vi "运维调试_氨氮.vi"() -> ()   [LabVIEW 2016, in "氨氮.lvlib"]
uses:
  <vilib>/Platform/TimedLoop/XDataNode/timing_clust.ctl
  <vilib>/Platform/TimedLoop/XDataNode/nitl_modes.ctl
  <vilib>/Platform/TimedLoop/XDataNode/wakeup.ctl
  <vilib>/Utility/miscctls.llb/LVPointTypeDef.ctl
  <vilib>/Platform/TimedLoop/XDataNode/XDataNode.xnode
  <vilib>/Platform/TimedLoop/XDataNode/XDNodeRunTimeDep.lvlib
panel:
  out "固件版本号":string
  in  "数组":string[](array[string])
  in  "备用系数写入":bool
  in  "备用系数读取":bool
  in  "备用系数":T1
  in  "量程切换阈值写入":bool
  in  "量程切换阈值读取":bool
  in  "量程切换阈值":cluster{"阈值":dbl, "标液浓度":dbl}
  in  "参数下拉列表":enum16{"氨氮", "总磷"}(ring)
  in  "量程下拉列表":enum16{"低量程", "高量程"}(ring)
  in  "测量模式下拉列表":enum16{"水样测量", "空白核查", "标样核查", "盲样测试", "加标回收"}(ring)
  in  "公式":cluster{"X^2":dbl, "X":dbl, "b":dbl}
  in  "写公式":bool
  in  "读公式":bool
  in  "精度":dbl=4.0
  in  "样品5 F0":dbl
  in  "样品5 F1":dbl
  in  "样品4 F1":dbl
  in  "样品4 F0":dbl
  in  "样品3 F0":dbl
  in  "样品3 F1":dbl
  in  "样品2 F0":dbl
  in  "样品2 F1":dbl
  in  "样品1 F1":dbl
  in  "样品1 F0":dbl
  in  "method":u16(ring) items=["最小二乘", "最小绝对残差", "Bisquare"]
  in  "模型":enum32{"线性", "多项式"}(ring)
  out "r^2":dbl format="%.7g"
  out "拟合公式":string
  in  "样品2启用":bool
  in  "样品5启用":bool
  in  "样品4启用":bool
  in  "样品3启用":bool
  in  "样品1启用":bool
  in  "标液浓度5":dbl
  out "测量吸光度5":dbl
  in  "标液浓度4":dbl
  out "测量吸光度4":dbl
  in  "标液浓度3":dbl
  out "测量吸光度3":dbl
  in  "标液浓度2":dbl
  out "测量吸光度2":dbl
  out "测量吸光度1":dbl
  in  "标液浓度1":dbl
  out "XY图":cluster{"X Values":dbl[], "Y Values":dbl[]}[](graph)
  in  "返回":bool
  in  "设置":bool
  out "序列号":string="序列号"
  out "氨氮测量数据":T2(xcontrol)
  out "集成报警信息":string
  out "设置值":dbl
  out "定时启动":bool
  out "总磷总氮运行状态":T3(xcontrol)
  in  "停止":bool
  in  "手动启动":bool
  in  "单步测试":bool
  in  "总磷氨氮调试":u16[](xcontrol)
  out "F3":sgl format="%#.6f"
  out "F2":sgl format="%#.6f"
  out "F1":sgl format="%#.6f"
  out "F0":sgl format="%#.6f"
  out "多列列表框":i32(listbox)
  # "COM7"
  # "参数设置"
  # "标液浓度"
  # "F0"
  # "F1"
  # "吸光值显示"
  # "样品一"
  # "辅\n助\n计\n算\n区"
  # "样品二"
  # "样品三"
  # "样品四"
  # "样品五"
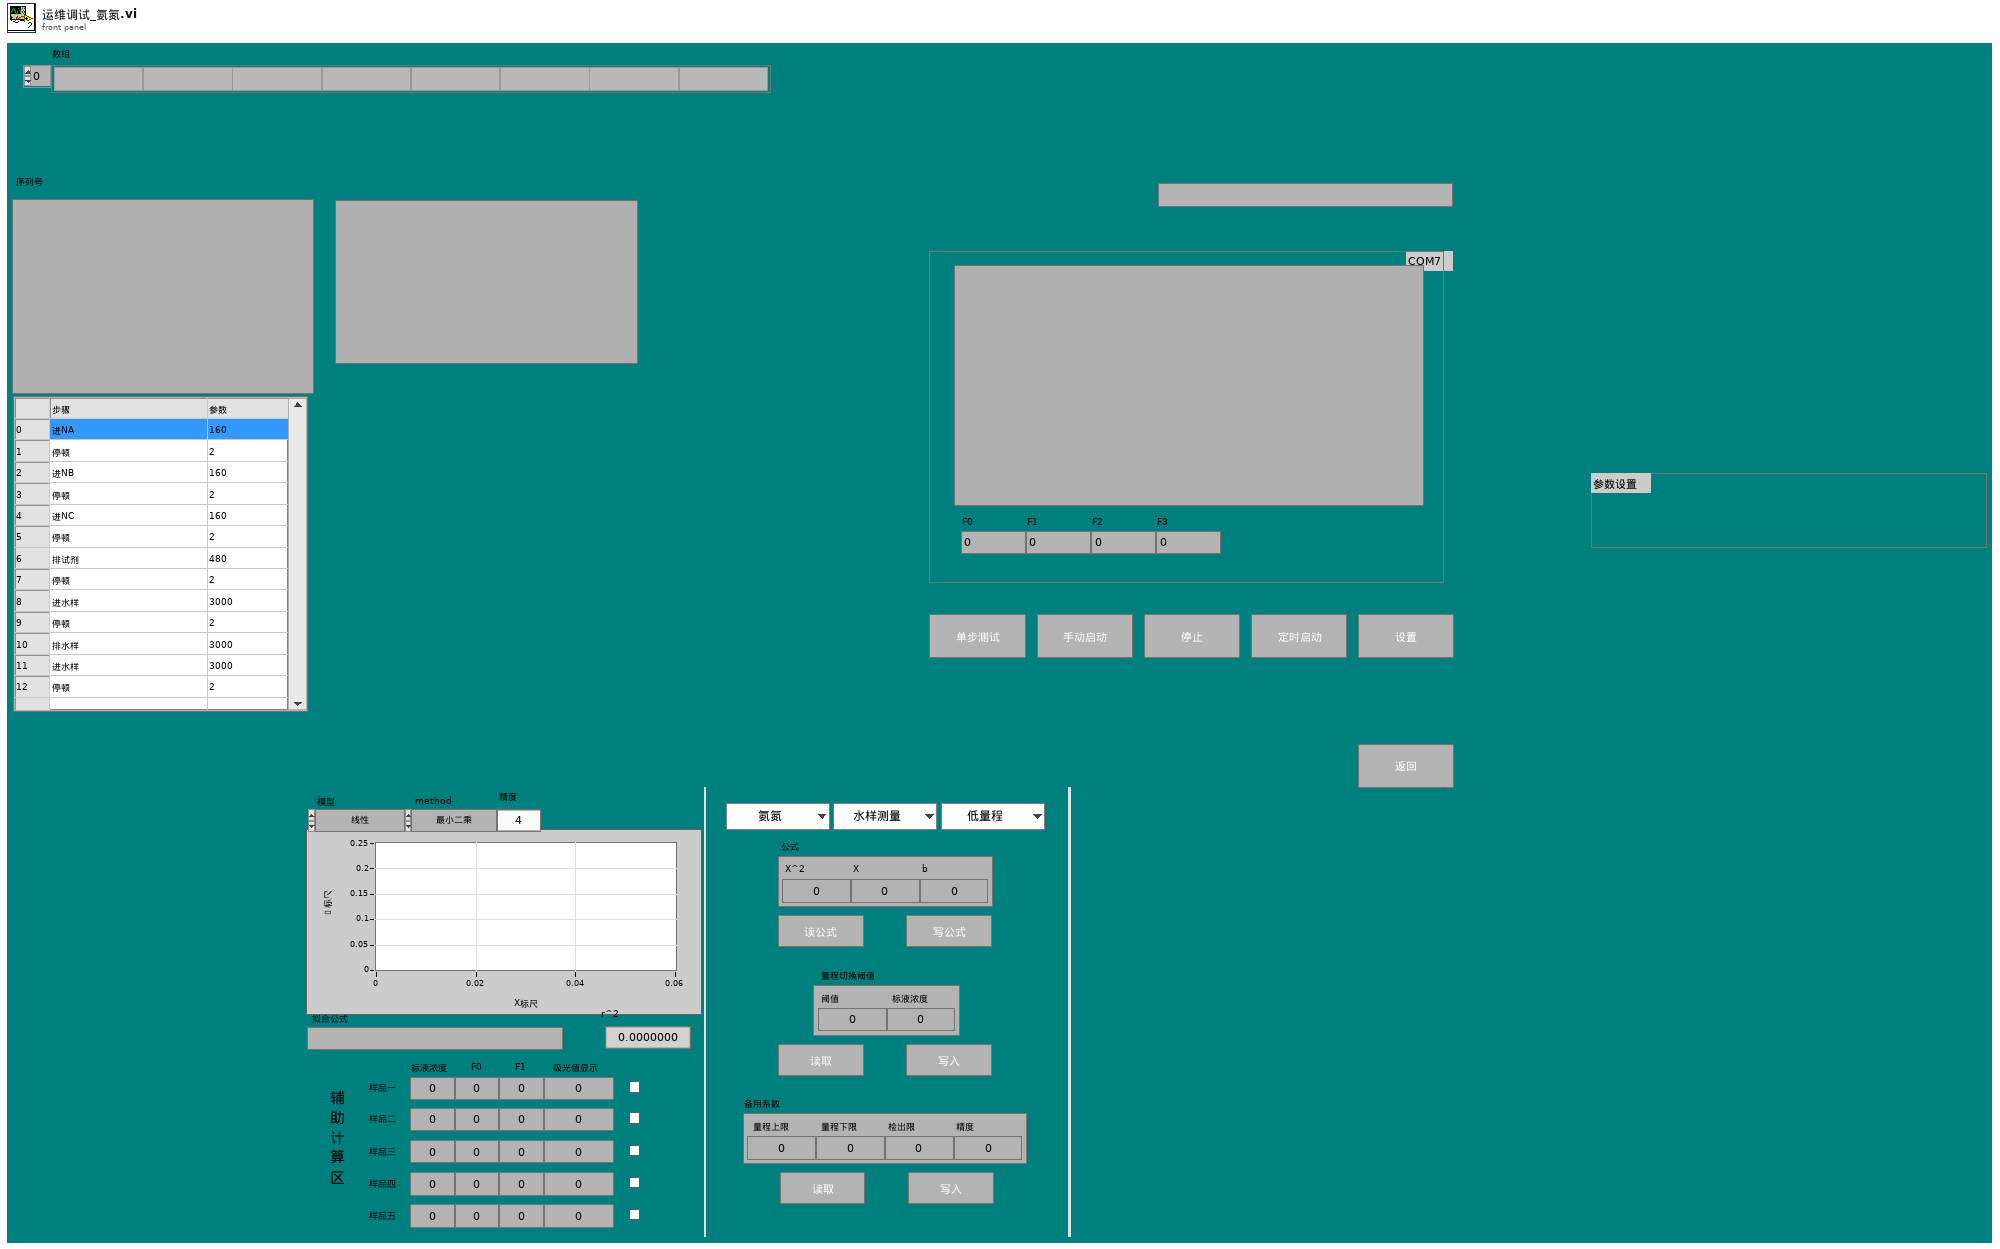
[diagram p1: front panel]
types:
  T1 = cluster{"量程上限":dbl, "量程下限":dbl, "检出限":dbl, "精度":dbl}
  T2 = cluster{"flowid":u16, "测量精度":u16, "测量数据区":cluster{"因子编码":u32, "单位":u16, "标样参考值":sgl, "水样数据时间":timestamp, "水样实测值":sgl, "水样数据标识":string, "标样数据时间":timestamp, "标样实测值":sgl, "标样数据标识":string, "空白数据时间":timestamp, "空白实测值":sgl, "空白数据标识":string, "零点核查数据时间":timestamp, "零点核查实测值":sgl, "零点核查数据标识":string, "跨度核查数据时间":timestamp, "跨度核查实测值":sgl, "跨度核查数据标识":string, "加标回收数据时间":timestamp, "加标回收实测值":sgl, "加标回收数据标识":string, "平行样数据时间":timestamp, "平行样实测值":sgl, "平行样数据标识":string}}
  T3 = cluster{"系统时间":timestamp, "工作状态":enum16{"空闲", "水样测试", "标样核查", "零点核查", "跨度核查", "空白测试", "平行样测试", "加标回收", "空白校准", "标样校准", "初始化（清洗）"}, "测量模式":enum16{"待机", "连续模式", "周期模式", "定点模式", "受控模式", "手动模式"}, "告警代码":enum16{"无告警", "缺试剂告警", "缺水样告警", "缺蒸馏水告警", "缺标液告警", "仪表漏液告警", "标定异常告警", "超量程告警", "加热异常", "低试剂预警", "超上限告警", "超下限告警", "仪表内部其他异常", "滴定异常告警", "电极异常告警", "量程切换告警", "参数设置告警", "PH电极电位异常", "电导率电极异常", "浊度光度异常", "溶解氧电极异常", "溶解氧光强异常", "温度异常告警", "PH异常告警", "溶解氧异常告警", "电导率异常告警", "浊度异常告警", "叶绿素异常告警", "藻密度异常告警", "蓝绿藻异常告警", "ORP异常告警", "氨氮异常告警", "清洁刷异常告警", "SD卡异常告警", "蓝牙异常告警", "Wifi异常告警", "流程异常告警"}, "故障代码":enum16{"无故障", "电机故障", "温度故障", "通讯故障", "滴定故障"}, "日志代码":u16, "软件版本":u16, "F0":sgl, "F1":sgl, "F2":sgl, "F3":sgl, "T":sgl, "H":sgl, "id":u16, "flowid":u16, "量程":u16}
  T4 = enum16{"待机", "启动氨氮", "氨氮测量中", "启动总磷", "总磷测量中", "延时"}
  T5 = typedef "LVPointTypeDef.ctl" = cluster{"Horizontal":i16, "Vertical":i16}
  T6 = cluster{"因子编码":u32, "单位":u16, "标样参考值":sgl, "水样数据时间":timestamp, "水样实测值":sgl, "水样数据标识":string, "标样数据时间":timestamp, "标样实测值":sgl, "标样数据标识":string, "空白数据时间":timestamp, "空白实测值":sgl, "空白数据标识":string, "零点核查数据时间":timestamp, "零点核查实测值":sgl, "零点核查数据标识":string, "跨度核查数据时间":timestamp, "跨度核查实测值":sgl, "跨度核查数据标识":string, "加标回收数据时间":timestamp, "加标回收实测值":sgl, "加标回收数据标识":string, "平行样数据时间":timestamp, "平行样实测值":sgl, "平行样数据标识":string}
  T7 = enum16{"空闲", "水样测试", "标样核查", "零点核查", "跨度核查", "空白测试", "平行样测试", "加标回收", "空白校准", "标样校准", "初始化（清洗）"}
  T8 = cluster{"启动模式":enum16{"标液测量", "水样测量", "零液测量", "盲样测量", "加标回收"}, "启动参数":u16, "量程":enum16{"低量程", "高量程"}}
  T9 = cluster{"时间标识":timestamp, "设备":string, "日志信息":string, "流程参数":string}
  T10 = cluster{"时间标识":timestamp, "设备":string, "日志信息":string}
  T11 = enum16{"无告警", "缺试剂告警", "缺水样告警", "缺蒸馏水告警", "缺标液告警", "仪表漏液告警", "标定异常告警", "超量程告警", "加热异常", "低试剂预警", "超上限告警", "超下限告警", "仪表内部其他异常", "滴定异常告警", "电极异常告警", "量程切换告警", "参数设置告警", "PH电极电位异常", "电导率电极异常", "浊度光度异常", "溶解氧电极异常", "溶解氧光强异常", "温度异常告警", "PH异常告警", "溶解氧异常告警", "电导率异常告警", "浊度异常告警", "叶绿素异常告警", "藻密度异常告警", "蓝绿藻异常告警", "ORP异常告警", "氨氮异常告警", "清洁刷异常告警", "SD卡异常告警", "蓝牙异常告警", "Wifi异常告警", "流程异常告警"}
  T12 = typedef "LVRowAndColumnUnsignedTypeDef.ctl" = cluster{"Row":u32, "Column":u32}
  T13 = typedef "XDNodeRunTimeDep.lvlib/timing_clust.ctl" = cluster{"Expected End [f-1]":u64, "Actual End [f-1]":u64, "Finished Late? [f-1]":bool, "Expected End [i-1]":u64, "Actual End [i-1]":u64, "Finished Late? [i-1]":bool, "Expected Start [i]":u64, "Actual Start [i]":u64, "Expected Start [f]":u64, "Actual Start [f]":u64, "Source Name":string, "Structure Name":string, "Period":i64, "Deadline":i64, "Offset":i64, "Start":i64, "Priority":i32, "Timeout":i32, "Mode":T14, "Wakeup Reason":T15, "Error":errorcluster, "Source Type":string, "Secondary Source Type":string, "Global End Time":u64, "Global Start Time":u64, "Frame Duration":u64, "Iteration Duration":u64, "Assigned CPU":i32, "I/O Scan Engine Mode":u32}
  T14 = typedef "XDNodeRunTimeDep.lvlib/nitl_modes.ctl" = enum32{"No Change", "Process missed periods, maintain original phase", "Discard missed periods, maintain original phase", "Process missed periods, ignore original phase", "Discard missed periods, ignore original phase"}
  T15 = typedef "XDNodeRunTimeDep.lvlib/wakeup.ctl" = enum32{"Normal", "Aborted", "Asynchronous wakeup", "Timing source error", "Timed loop error", "Timeout"}
  T16 = cluster{"站号":u16, "量程切换":enum32{"H", "L", "AUTO"}, "控制命令":enum16{"启动测量", "标样核查", "零点核查", "跨度核查", "空白测试", "平行样测试", "加标回收", "空白校准", "标样校准", "初始化（清洗）", "停止测试", "仪器重启", "校时", "模式设置", "测量间隔设置", "盲样测试"}, "模式设置":enum16{"待机", "连续模式", "周期模式", "定点模式", "受控模式", "手动模式"}, "测量间隔":u16}
  T17 = cluster{"站号":u16, "量程切换":enum32{"H", "L", "AUTO"}, "控制命令":enum16{"启动测量", "标样核查", "零点核查", "跨度核查", "空白测试", "平行样测试", "加标回收", "空白校准", "标样校准", "初始化（清洗）", "停止测试", "仪器重启", "校时", "模式设置", "测量间隔设置"}, "模式设置":enum16{"待机", "连续模式", "周期模式", "定点模式", "受控模式", "手动模式"}, "测量间隔":u16}
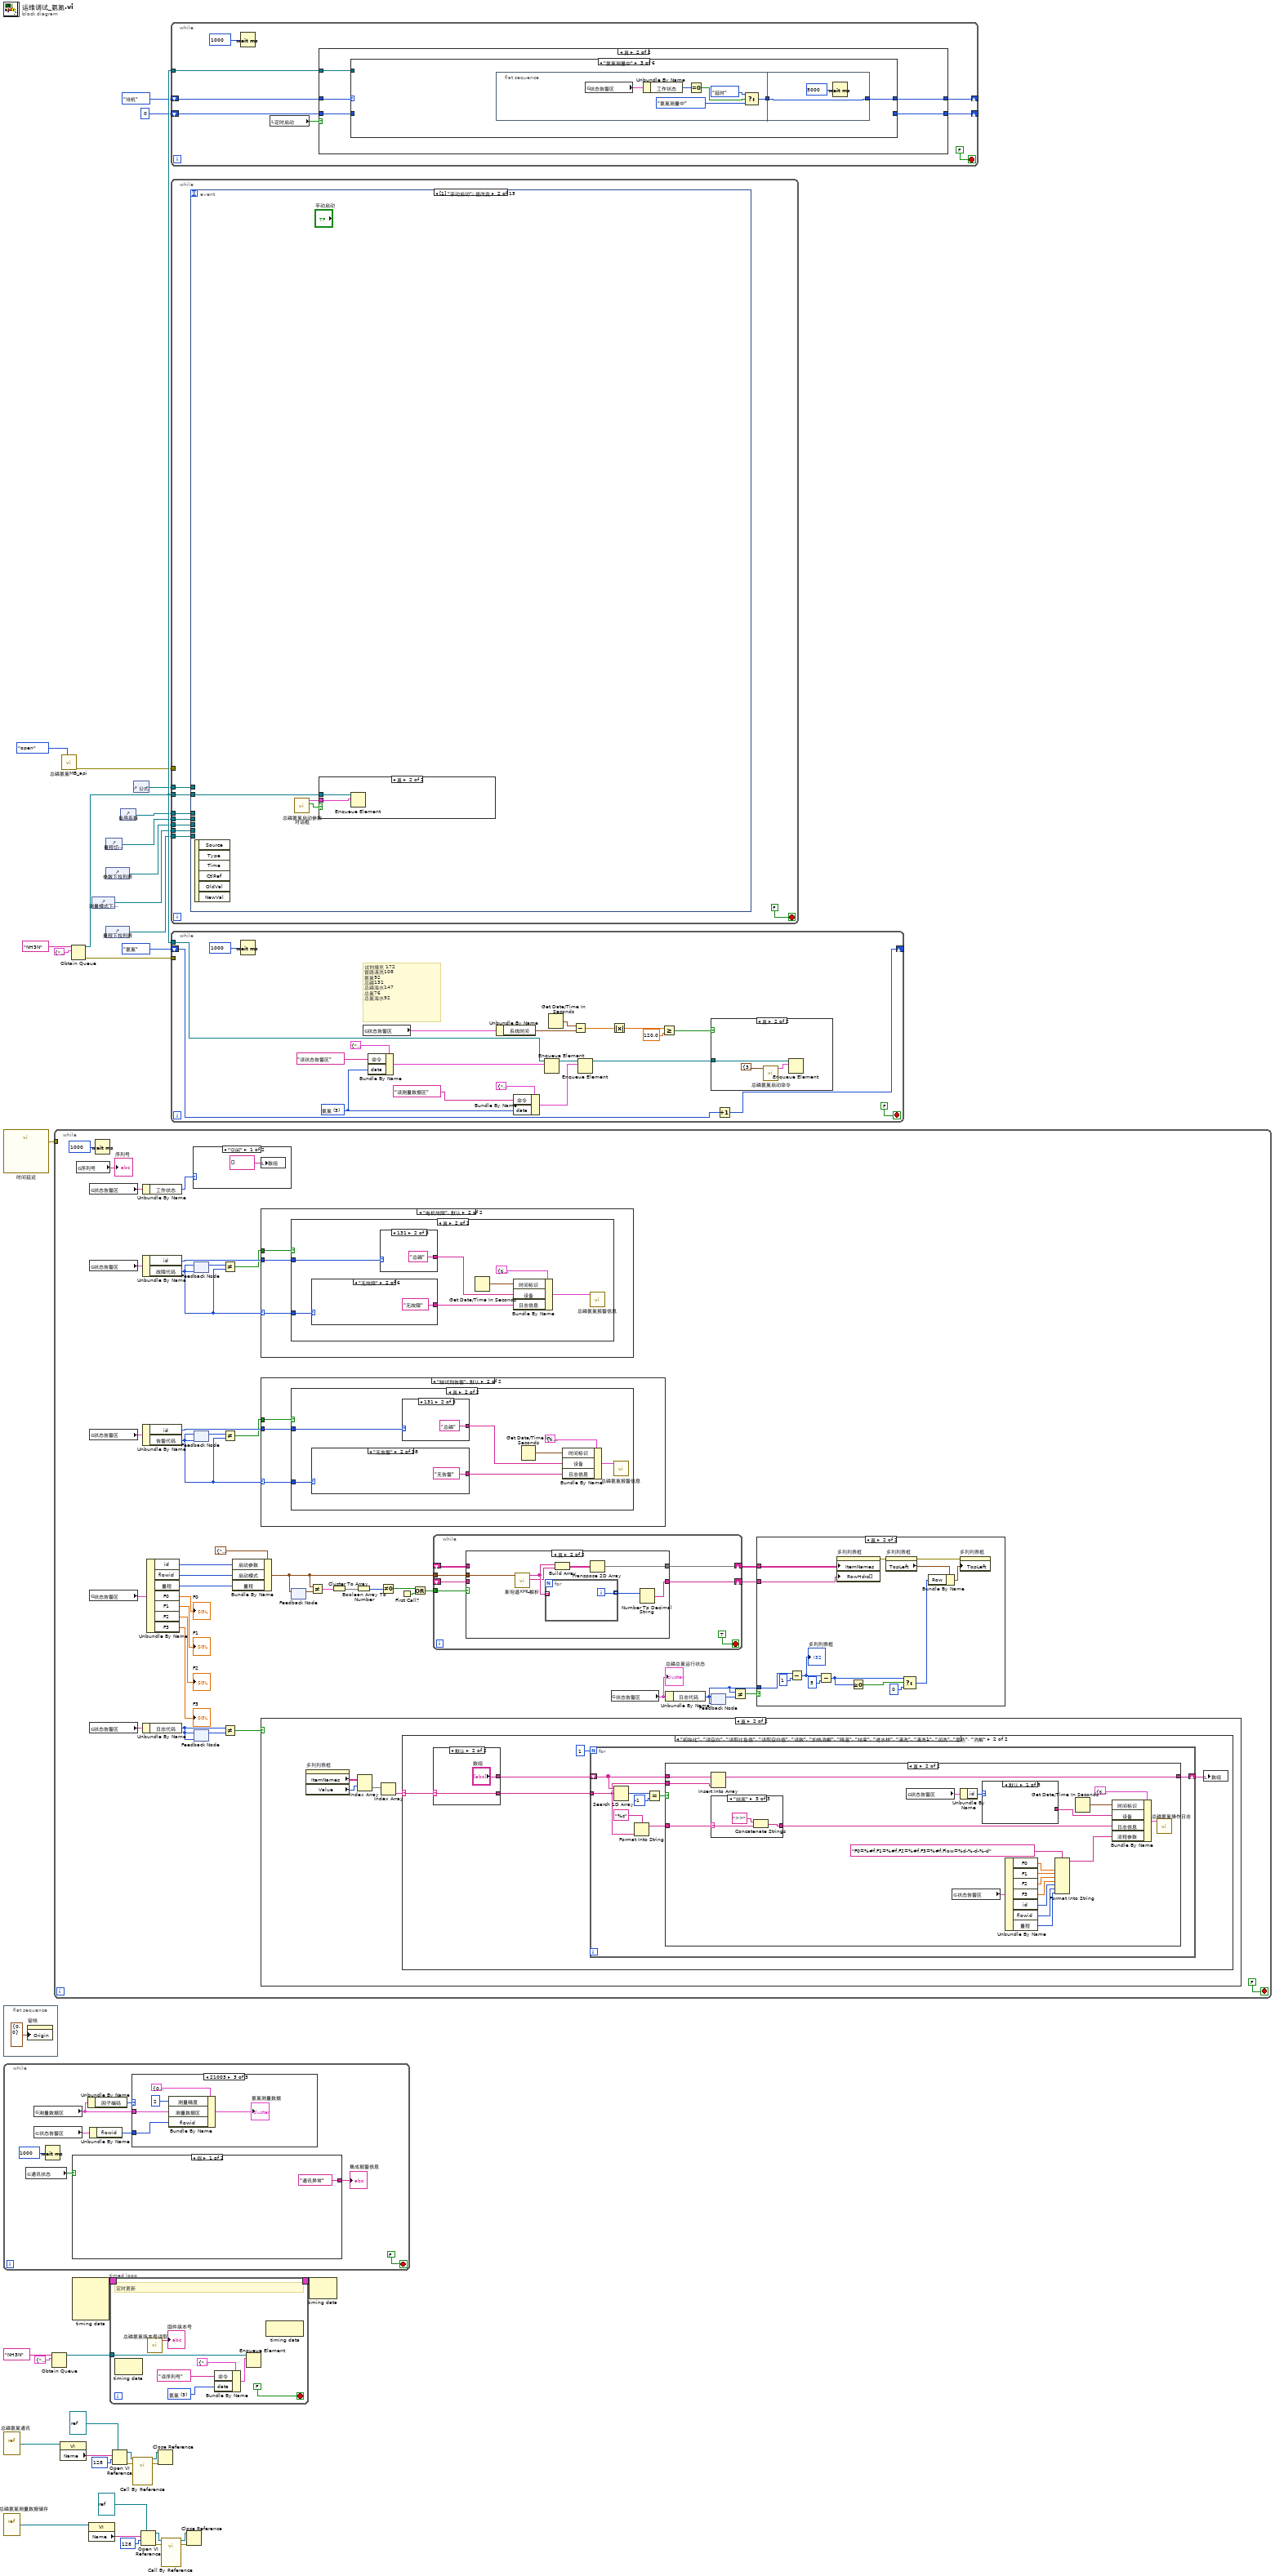
[diagram p0: block diagram]
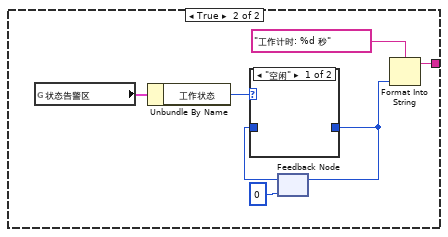
[diagram p2: hidden frame]
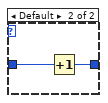
[diagram p3: hidden frame]
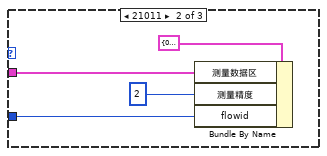
[diagram p5: hidden frame]
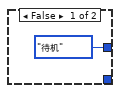
[diagram p6: hidden frame]
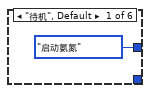
[diagram p7: hidden frame]
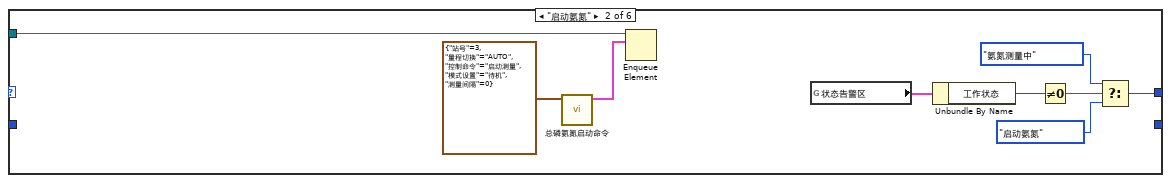
[diagram p8: hidden frame]
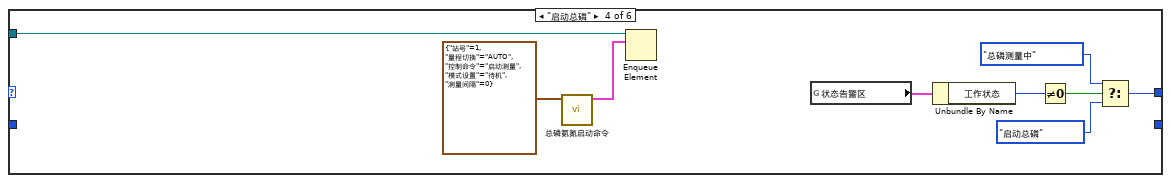
[diagram p9: hidden frame]
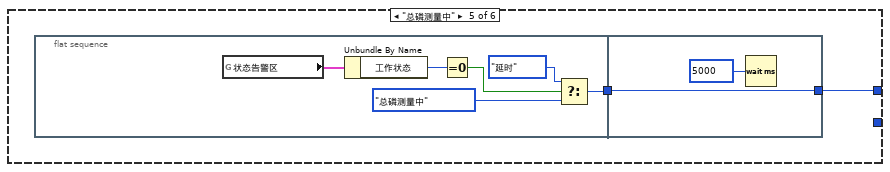
[diagram p10: hidden frame]
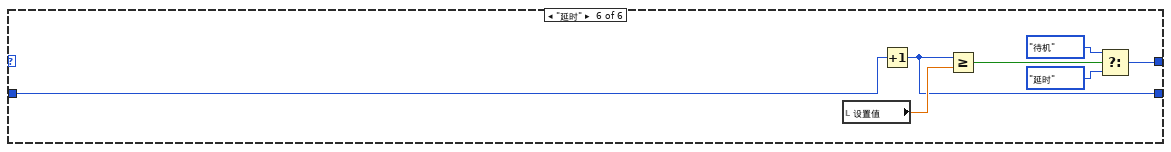
[diagram p11: hidden frame]
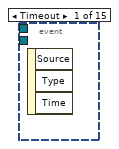
[diagram p12: hidden frame]
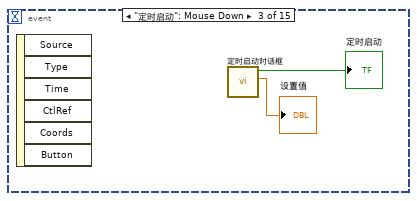
[diagram p14: hidden frame]
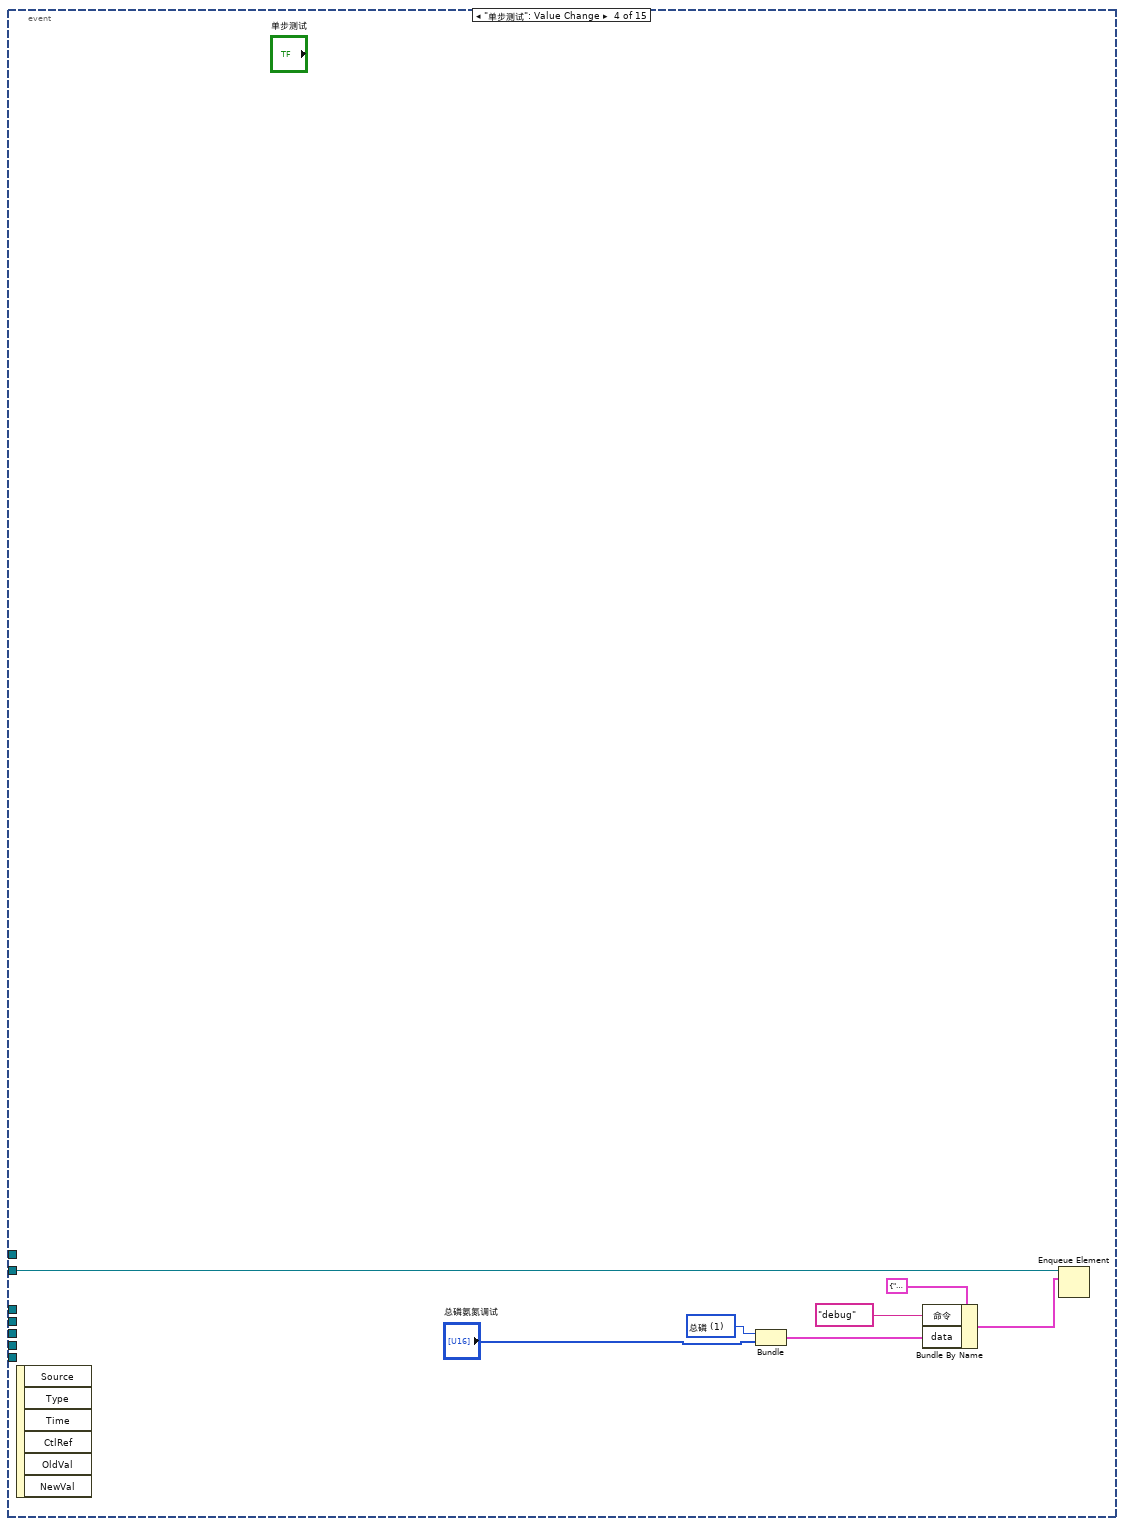
[diagram p15: hidden frame]
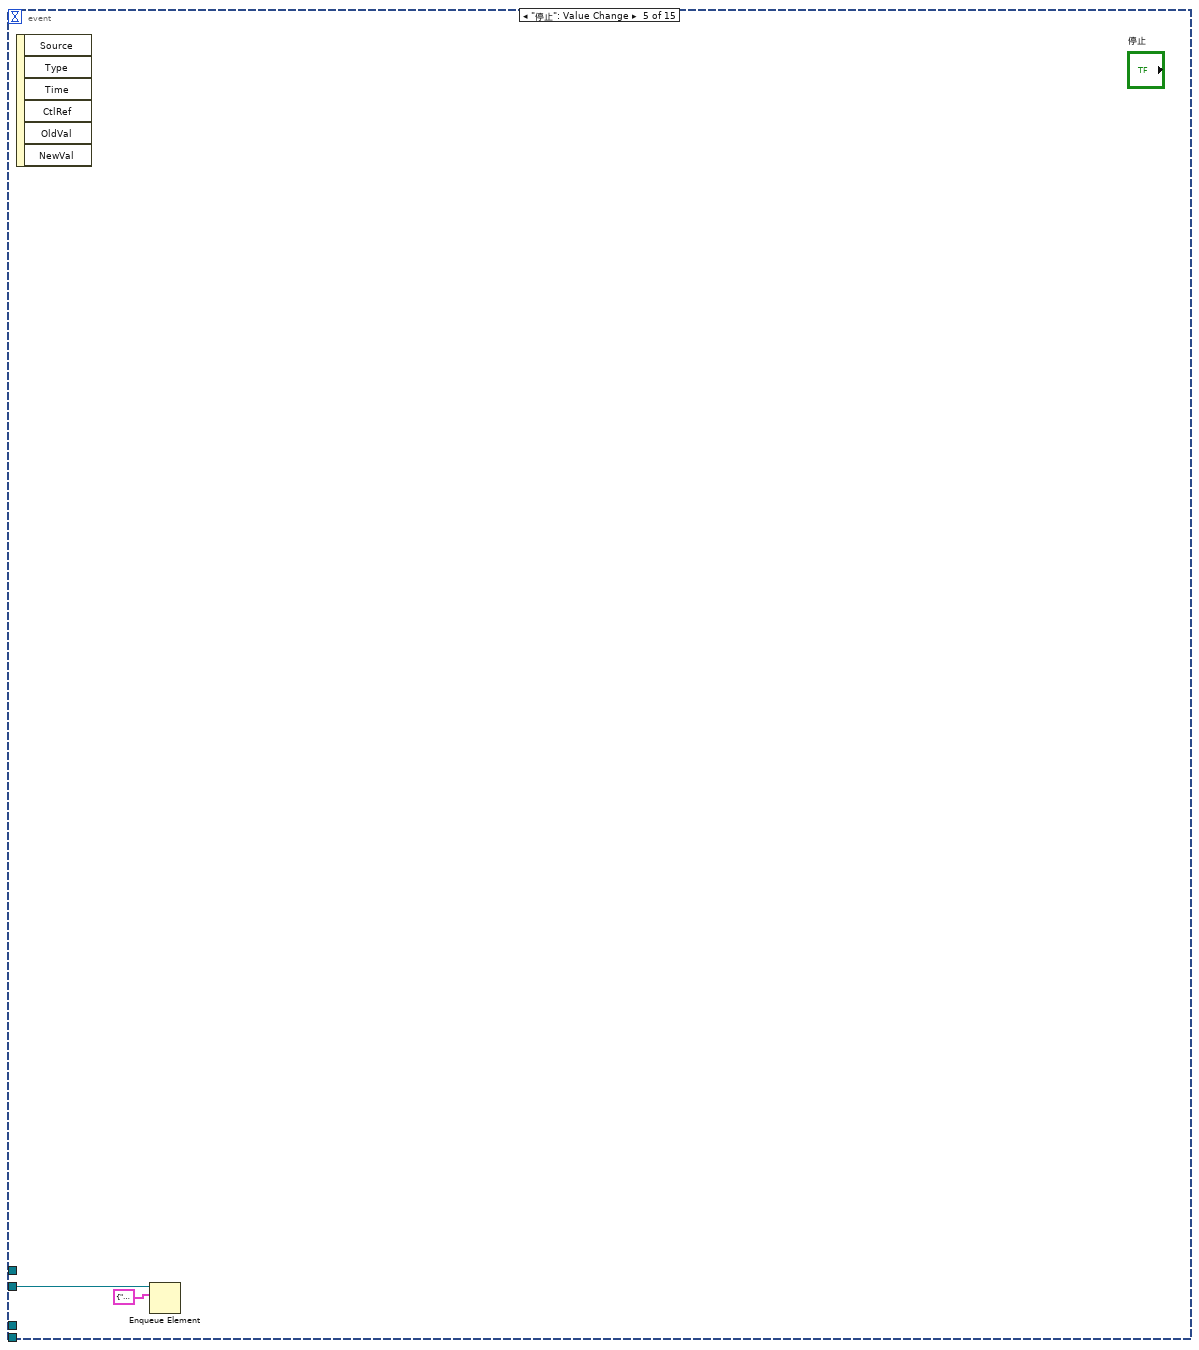
[diagram p16: hidden frame]
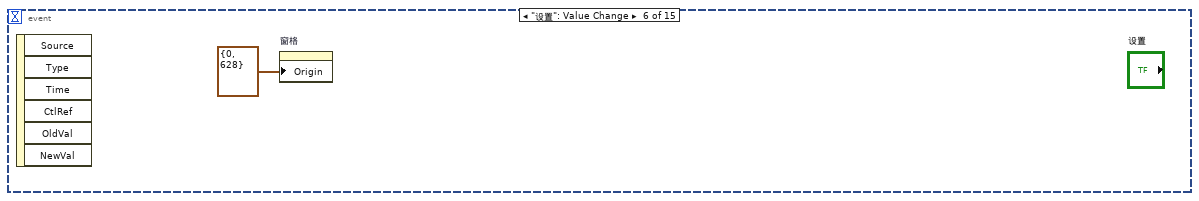
[diagram p17: hidden frame]
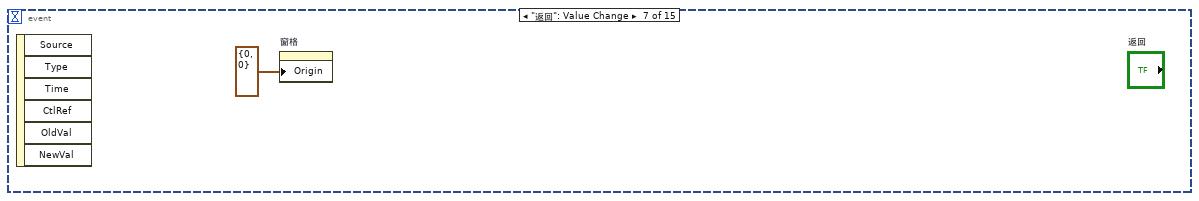
[diagram p18: hidden frame]
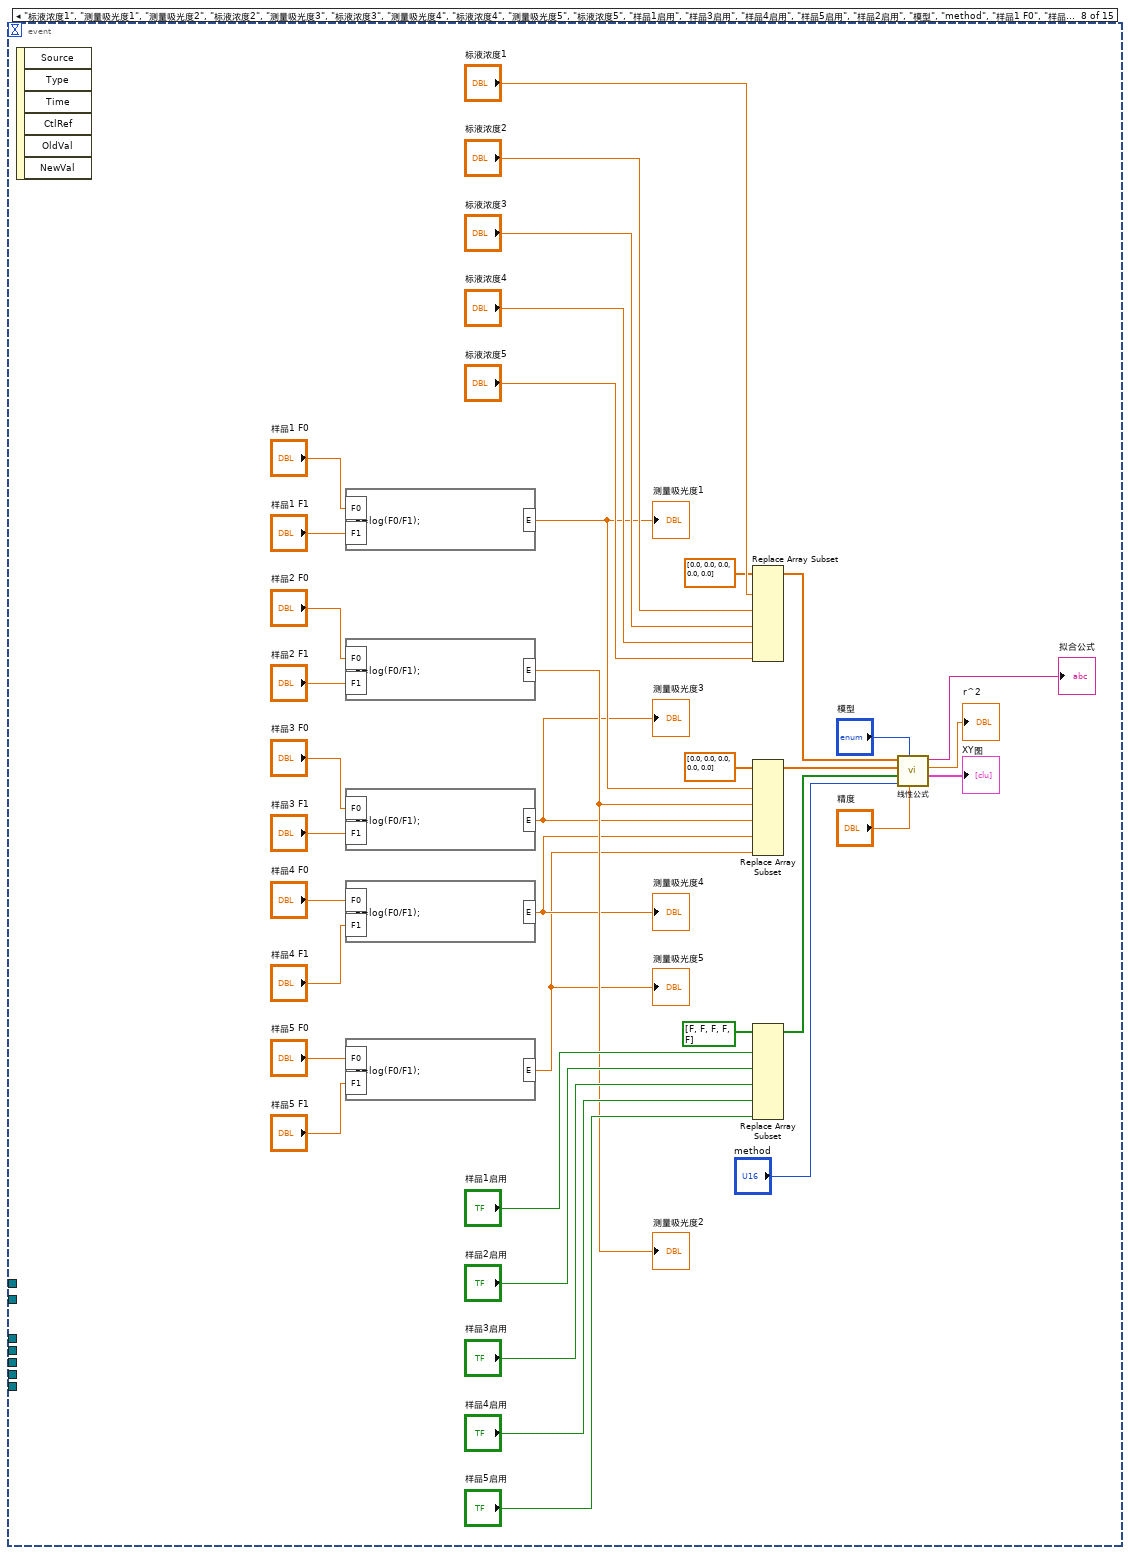
[diagram p19: hidden frame]
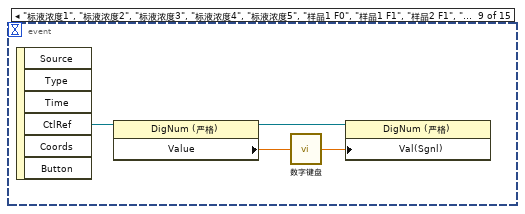
[diagram p20: hidden frame]
diagram:
  n1 = call "时间延迟"() -> ("error out"=w8:errorcluster)  [unwired: 11 in]
  n2 = flat-sequence {
    frame #0 {
      n3 = property on="窗格" class="Pane"("Origin"=T5 {"Horizontal"=0, "Vertical"=0} ("原点")) -> ()  [unwired: 2 in, 2 out]
    }
  }
  n4 = while {
    stop <- FALSE stop-if-true
    n5 = global read "VAR总磷氨氮全局变量.vi" "通讯状态"() -> (w42:bool)
    n6 = global read "VAR总磷氨氮全局变量.vi" "测量数据区"() -> (w44:T6)
    n7 = global read "VAR总磷氨氮全局变量.vi" "状态告警区"() -> (w40:T3)
    n8 = Wait (ms)(milliseconds to wait=u32 1000 ("等待时间（毫秒）")) -> ()  [unwired: 1 out]
    n9 = case shown="假" w42 {
      tunnel: ["通讯异常" ("集成报警信息") w48] -> w41
      frame False {
      }
      frame True {
        n10 = global read "VAR总磷氨氮全局变量.vi" "状态告警区"() -> (w54:T3)
        n11 = Unbundle By Name(w54) -> ("工作状态"=w53:T7)
        n12 = feedback #1(0) -> (w51:i32)
        n13 = case shown="\"空闲\"" w53 {
          tunnel: w51 -> [_ w56]
          tunnel: [_ w55] -> w49
          frame "空闲" {
          }
          frame Default {
            n14 = Increment(x=w56) -> (x+1=w55:i32)
          }
        }
        n15 = feedback-in #1(w49) -> ()
        n16 = Format Into String(format string="工作计时: %d 秒" ("格式字符串"), w49) -> (resulting string=w48:string)  [unwired: 2 in, 1 out]
      }
    }
    "集成报警信息" <- w41
    n17 = Unbundle By Name(w44) -> ("因子编码"=w43:u32)
    n18 = Unbundle By Name(w40) -> ("flowid"=w39:u16)
    n19 = case shown="21003" w43 {
      tunnel: w44 -> [_ w60 w65]
      tunnel: w39 -> [_ w58 w63]
      frame Default {
      }
      frame 21011 {
        n20 = Bundle By Name(cluster=T2 {"flowid"=0, "测量精度"=0, "测量数据区"={"因子编码"=0, "单位"=0, "标样参考值"=0.0, "水样数据时间"=timestamp(0 s since 1904-01-01), "水样实测值"=0.0, "水样数据标识"="", "标样数据时间"=timestamp(0 s since 1904-01-01), "标样实测值"=0.0, "标样数据标识"="", "空白数据时间"=timestamp(0 s since 1904-01-01), "空白实测值"=0.0, "空白数据标识"="", "零点核查数据时间"=timestamp(0 s since 1904-01-01), "零点核查实测值"=0.0, "零点核查数据标识"="", "跨度核查数据时间"=timestamp(0 s since 1904-01-01), "跨度核查实测值"=0.0, "跨度核查数据标识"="", "加标回收数据时间"=timestamp(0 s since 1904-01-01), "加标回收实测值"=0.0, "加标回收数据标识"="", "平行样数据时间"=timestamp(0 s since 1904-01-01), "平行样实测值"=0.0, "平行样数据标识"=""}} ("氨氮测量数据"), "测量数据区"=w60, "测量精度"=u16 2, "flowid"=w58) -> ()  [unwired: 1 out]
      }
      frame 21003 {
        n21 = Bundle By Name(cluster=T2 {"flowid"=0, "测量精度"=0, "测量数据区"={"因子编码"=0, "单位"=0, "标样参考值"=0.0, "水样数据时间"=timestamp(0 s since 1904-01-01), "水样实测值"=0.0, "水样数据标识"="", "标样数据时间"=timestamp(0 s since 1904-01-01), "标样实测值"=0.0, "标样数据标识"="", "空白数据时间"=timestamp(0 s since 1904-01-01), "空白实测值"=0.0, "空白数据标识"="", "零点核查数据时间"=timestamp(0 s since 1904-01-01), "零点核查实测值"=0.0, "零点核查数据标识"="", "跨度核查数据时间"=timestamp(0 s since 1904-01-01), "跨度核查实测值"=0.0, "跨度核查数据标识"="", "加标回收数据时间"=timestamp(0 s since 1904-01-01), "加标回收实测值"=0.0, "加标回收数据标识"="", "平行样数据时间"=timestamp(0 s since 1904-01-01), "平行样实测值"=0.0, "平行样数据标识"=""}} ("氨氮测量数据"), "测量精度"=u16 2, "测量数据区"=w65, "flowid"=w63) -> (→"氨氮测量数据":T2)
      }
    }
  }
  n22 = vi-ref "总磷氨氮通讯.vi"() -> (w31:refnum<vi>)
  n23 = vi-ref "总磷氨氮测量数据储存.vi"() -> (w23:refnum<vi>)
  n24 = Obtain Queue(name (unnamed)="NH3N" ("名称（未命名）"), element data type=cluster{"命令":string, "data":variant} {"命令"="", "data"=variant}) -> (queue out=w1:refnum<queue>)  [unwired: 3 in, 2 out]
  n25 = while {
    tunnel: w8 -> [_]
    stop <- FALSE stop-if-true
    n26 = global read "VAR总磷氨氮全局变量.vi" "序列号"() -> (→"序列号":string)
    n27 = global read "VAR总磷氨氮全局变量.vi" "状态告警区"() -> (w71:T3)
    n28 = global read "VAR总磷氨氮全局变量.vi" "状态告警区"() -> (w77:T3)
    n29 = global read "VAR总磷氨氮全局变量.vi" "状态告警区"() -> (w82:T3)
    n30 = global read "VAR总磷氨氮全局变量.vi" "状态告警区"() -> (w94:T3)
    n31 = global read "VAR总磷氨氮全局变量.vi" "状态告警区"() -> (w68:T3)
    n32 = Wait (ms)(milliseconds to wait=u32 1000 ("等待时间（毫秒）")) -> ()  [unwired: 1 out]
    n33 = Unbundle By Name(w71) -> ("工作状态"=w70:T7)
    n34 = Unbundle By Name(w77) -> ("id"=w76:u16, "故障代码"=w73:enum16{"无故障", "电机故障", "温度故障", "通讯故障", "滴定故障"})
    n35 = Unbundle By Name(w82) -> ("id"=w81:u16, "告警代码"=w78:T11)
    n36 = Unbundle By Name(w68) -> ("日志代码"=w67:u16)
    n37 = Unbundle By Name(w94) -> ("id"=w91:u16, "flowid"=w93:u16, "量程"=w92:u16, "F0"=→"F0":sgl, "F1"=→"F1":sgl, "F2"=→"F2":sgl, "F3"=→"F3":sgl)
    n38 = case shown="\"空闲\"" w70 {
      frame "空闲" {
        n39 = local write "数组"(string[] [] ("数组")) -> ()
      }
      frame "水样测试", Default {
      }
    }
    n40 = feedback #2(w73) -> (w74:enum16{"无故障", "电机故障", "温度故障", "通讯故障", "滴定故障"})
    n41 = feedback-in #2(w73) -> ()
    n42 = feedback #3(w78) -> (w79:T11)
    n43 = feedback-in #3(w78) -> ()
    n44 = feedback #4(w67) -> (w69:u16)
    n45 = feedback-in #4(w67) -> ()
    n46 = Not Equal?(x=w74, y=w73) -> (x != y?=w75:bool)
    n47 = Not Equal?(x=w79, y=w78) -> (x != y?=w80:bool)
    n48 = Not Equal?(x=w67, y=w69) -> (x != y?=w66:bool)
    n49 = Bundle By Name(cluster=T8 {"启动模式"=enum."加标回收", "启动参数"=1, "量程"=enum."低量程"} ("参数簇"), "启动参数"=w91, "启动模式"=w93, "量程"=w92) -> (w84:T8)
    n50 = case shown="\"电机故障\", 默认" w73 {
      selector: w73 -> [_ w162]
      tunnel: w76 -> [_ w163]
      tunnel: w75 -> [_ w161]
      frame "无故障" {
      }
      frame "电机故障", Default {
        n51 = case shown="真" w161 {
          tunnel: w163 -> [_ w170]
          tunnel: w162 -> [_ w165]
          frame False {
          }
          frame True {
            n52 = case shown="\"无故障\"" w165 {
              selector: w165 -> [w172 _ _ _ _ _]
              tunnel: [w171 "无故障" "电机故障" "温度故障" "通讯故障" "滴定故障"] -> w164
              frame Default {
                n53 = Format Into String(format string="%d" ("格式字符串"), initial string="未知" ("工作状态"), w172) -> (resulting string=w171:string)  [unwired: 1 in, 1 out]
              }
              frame "无故障" {
              }
              frame "电机故障" {
              }
              frame "温度故障" {
              }
              frame "通讯故障" {
              }
              frame "滴定故障" {
              }
            }
            n54 = case shown="131" w170 {
              tunnel: [_ "总磷" ("table输入") "氨氮" ("table输入")] -> w166
              frame Default {
              }
              frame 131 {
              }
              frame 92 {
              }
            }
            n55 = Get Date/Time In Seconds() -> (seconds since 1Jan1904=w167:timestamp)
            n56 = Bundle By Name(cluster=T10 {"时间标识"=timestamp(0 s since 1904-01-01), "设备"="", "日志信息"=""} ("data in"), "时间标识"=w167, "设备"=w166, "日志信息"=w164) -> (w168:T10)
            n57 = call "总磷氨氮报警信息.vi"("data in"=w168) -> ()  [unwired: 11 in]
          }
        }
      }
    }
    n58 = case shown="\"缺试剂告警\", 默认" w78 {
      selector: w78 -> [_ w183]
      tunnel: w81 -> [_ w184]
      tunnel: w80 -> [_ w182]
      frame "无告警" {
      }
      frame "缺试剂告警", Default {
        n59 = case shown="真" w182 {
          tunnel: w184 -> [_ w191]
          tunnel: w183 -> [_ w185]
          frame False {
          }
          frame True {
            n60 = case shown="\"无告警\"" w185 {
              selector: w185 -> [w193 _ _ _ _ _ _ _ _ _ _ _ _ _ _ _ _ _ _ _ _ _ _ _ _ _ _ _ _ _ _ _ _ _ _ _ _ _]
              tunnel: [w192 "无告警" "缺试剂告警" "缺水样告警" "缺蒸馏水告警" "缺标液告警" "仪表漏液告警" "标定异常告警" "超量程告警" "加热异常" "低试剂预警" "超上限告警" "超下限告警" "仪表内部其他异常" "滴定异常告警" "电极异常告警" "量程切换告警" "参数设置告警" "PH电极电位异常" "电导率电极异常" "浊度光度异常" "溶解氧电极异常" "溶解氧光强异常" "温度异常告警" "PH异常告警" "溶解氧异常告警" "电导率异常告警" "浊度异常告警" "叶绿素异常告警" "藻密度异常告警" "蓝绿藻异常告警" "ORP异常告警" "氨氮异常告警" "清洁刷异常告警" "SD卡异常告警" "蓝牙异常告警" "WiFi异常告警" "流程异常告警"] -> w186
              frame Default {
                n61 = Format Into String(format string="%d" ("格式字符串"), initial string="未知" ("工作状态"), w193) -> (resulting string=w192:string)  [unwired: 1 in, 1 out]
              }
              frame "无告警" {
              }
              frame "缺试剂告警" {
              }
              frame "缺水样告警" {
              }
              frame "缺蒸馏水告警" {
              }
              frame "缺标液告警" {
              }
              frame "仪表漏液告警" {
              }
              frame "标定异常告警" {
              }
              frame "超量程告警" {
              }
              frame "加热异常" {
              }
              frame "低试剂预警" {
              }
              frame "超上限告警" {
              }
              frame "超下限告警" {
              }
              frame "仪表内部其他异常" {
              }
              frame "滴定异常告警" {
              }
              frame "电极异常告警" {
              }
              frame "量程切换告警" {
              }
              frame "参数设置告警" {
              }
              frame "PH电极电位异常" {
              }
              frame "电导率电极异常" {
              }
              frame "浊度光度异常" {
              }
              frame "溶解氧电极异常" {
              }
              frame "溶解氧光强异常" {
              }
              frame "温度异常告警" {
              }
              frame "PH异常告警" {
              }
              frame "溶解氧异常告警" {
              }
              frame "电导率异常告警" {
              }
              frame "浊度异常告警" {
              }
              frame "叶绿素异常告警" {
              }
              frame "藻密度异常告警" {
              }
              frame "蓝绿藻异常告警" {
              }
              frame "ORP异常告警" {
              }
              frame "氨氮异常告警" {
              }
              frame "清洁刷异常告警" {
              }
              frame "SD卡异常告警" {
              }
              frame "蓝牙异常告警" {
              }
              frame "Wifi异常告警" {
              }
              frame "流程异常告警" {
              }
            }
            n62 = case shown="131" w191 {
              tunnel: [_ "总磷" ("table输入") "氨氮" ("table输入")] -> w187
              frame Default {
              }
              frame 131 {
              }
              frame 92 {
              }
            }
            n63 = Get Date/Time In Seconds() -> (seconds since 1Jan1904=w188:timestamp)
            n64 = Bundle By Name(cluster=T10 {"时间标识"=timestamp(0 s since 1904-01-01), "设备"="", "日志信息"=""} ("data in"), "时间标识"=w188, "设备"=w187, "日志信息"=w186) -> (w189:T10)
            n65 = call "总磷氨氮报警信息.vi"("data in"=w189) -> ()  [unwired: 11 in]
          }
        }
      }
    }
    n66 = case shown="真" w66 {
      frame False {
      }
      frame True {
        n67 = property on="多列列表框" class="MCListbox (严格)"() -> ("ItemNames"=w111:string[][], "Value"=w112:i32)  [unwired: 2 in, 2 out]
        n68 = Index Array(array=w111, index (row)=w112) -> (element=w110:string[])  [unwired: 1 in]
        n69 = Index Array(array=w110) -> (element=w109:string)  [unwired: 1 in]
        n70 = case shown="\"初始化\", \"读空白\", \"读取比色值\", \"读取空白值\", \"读数\", \"加热消解\", \"降温\", \"结束\", \"进水样\", \"清洗\", \"清洗1\", \"润洗\", \"显色\", \"消解\"" w109 {
          selector: w109 -> [_ w115]
          frame Default {
          }
          frame "初始化", "读空白", "读取比色值", "读取空白值", "读数", "加热消解", "降温", "结束", "进水样", "清洗", "清洗1", "润洗", "显色", "消解" {
            n71 = case shown="默认" w115 {
              selector: w115 -> [w119 w121]
              tunnel: [w119 w121] -> w114
              tunnel: [string[] [] ("数组") "数组"] -> w113
              frame "读数" {
              }
              frame Default {
              }
            }
            n72 = for {
              N: 1 -> [_]
              tunnel: w114 -> [w123]
              shift-right: [w122] -> w116
              shift-left: w113 -> [w124]
              n73 = Search 1D Array(1D array=w124, element=w123) -> (index of element=w127:i32)  [unwired: 1 in]
              n74 = Format Into String(format string="%s" ("格式字符串"), w123) -> (resulting string=w128:string)  [unwired: 2 in, 1 out]
              n75 = Equal?(x=w127, y=-1) -> (x = y?=w125:bool)
              n76 = case shown="真" w125 {
                tunnel: w128 -> [_ w132]
                tunnel: w124 -> [w130 w136]
                tunnel: w123 -> [_ w135]
                tunnel: [w130 w134] -> w122
                frame False {
                }
                frame True {
                  n77 = Insert Into Array(array=w136, new element=w135) -> (w134:string[])  [unwired: 1 in]
                  n78 = case shown="\"结束\"" w132 {
                    selector: w132 -> [w152 w155 w158]
                    tunnel: [w152 w154 w157] -> w131
                    frame Default {
                    }
                    frame "初始化" {
                      n79 = Concatenate Strings("<<" ("字符串"), w155) -> (w154:string)
                    }
                    frame "结束" {
                      n80 = Concatenate Strings(">>" ("字符串"), w158) -> (w157:string)
                    }
                  }
                  n81 = global read "VAR总磷氨氮全局变量.vi" "状态告警区"() -> (w151:T3)
                  n82 = global read "VAR总磷氨氮全局变量.vi" "状态告警区"() -> (w146:T3)
                  n83 = Unbundle By Name(w151) -> ("id"=w150:u16)
                  n84 = case shown="默认" w150 {
                    tunnel: [_ "总磷" ("table输入") "氨氮" ("table输入")] -> w148
                    frame Default {
                    }
                    frame 131 {
                    }
                    frame 92 {
                    }
                  }
                  n85 = Unbundle By Name(w146) -> ("F0"=w143:sgl, "F1"=w142:sgl, "F2"=w141:sgl, "F3"=w140:sgl, "id"=w139:u16, "flowid"=w138:u16, "量程"=w137:u16)
                  n86 = Format Into String(format string="F0=%#f,F1=%#f,F2=%#f,F3=%#f,Flow=%d-%-d-%-d" ("格式字符串"), w143, w142, w141, w140, w139, w138, w137) -> (resulting string=w144:string)  [unwired: 2 in, 1 out]
                  n87 = Get Date/Time In Seconds() -> (seconds since 1Jan1904=w147:timestamp)
                  n88 = Bundle By Name(cluster=T9 {"时间标识"=timestamp(0 s since 1904-01-01), "设备"="", "日志信息"="", "流程参数"=""} ("data in"), "时间标识"=w147, "设备"=w148, "日志信息"=w131, "流程参数"=w144) -> (w149:T9)
                  n89 = call "总磷氨氮操作日志.vi"("data in"=w149) -> ()  [unwired: 11 in]
                }
              }
            }
            n90 = local write "数组"(w116) -> ()
          }
        }
      }
    }
    n91 = feedback #5() -> (w100:T8)  [unwired: 1 in]
    n92 = feedback-in #5(w84) -> ()
    n93 = Not Equal?(x=w84, y=w100) -> (x != y?=w101:cluster{"启动模式":bool, "启动参数":bool, "量程":bool})
    n94 = Cluster To Array(cluster=w101) -> (array=w102:bool[])
    n95 = Boolean Array To Number(Boolean array=w102) -> (number=w103:u32)
    n96 = Not Equal To 0?(x=w103) -> (x != 0?=w96:bool)
    n97 = First Call?() -> (First Call?: T/F=w97:bool)
    n98 = Or(x=w96, y=w97) -> (x .or. y?=w95:bool)
    n99 = while {
      tunnel: w95 -> [w241]
      tunnel: w84 -> [w240]
      shift-right: [w239] -> w99
      shift-left: _ -> [w235]
      shift-right: [w238] -> w98
      shift-left: _ -> [w236]
      stop <- TRUE stop-if-true
      n100 = case shown="真" w241 {
        tunnel: [w243 w250] -> w238
        tunnel: [w242 w249] -> w239
        tunnel: w240 -> [_ w244]
        tunnel: w236 -> [w243 _]
        tunnel: w235 -> [w242 _]
        frame False {
        }
        frame True {
          n101 = call "斯坦道XML解析.vi"("参数簇"=w244) -> ("步骤时间"=w245:string[], "步骤名"=w247:string[])  [unwired: 9 in]
          n102 = for {
            tunnel: w247 -> [_] mode=indexing
            tunnel: [w251] -> w248 mode=indexing
            i -> [w251]
          }
          n103 = Build Array(w247, w245) -> (w246:string[][])
          n104 = Transpose 2D Array(2D array=w246) -> (transposed array=w249:string[][])
          n105 = Number To Decimal String(number=w248) -> (decimal integer string=w250:string[])  [unwired: 1 in]
        }
      }
    }
    n106 = global read "VAR总磷氨氮全局变量.vi" "状态告警区"() -> (w85:T3)
    "总磷总氮运行状态" <- w85
    n107 = Unbundle By Name(w85) -> ("日志代码"=w72:u16)
    n108 = feedback-in #6(w72) -> ()
    n109 = feedback #6(w72) -> (w105:u16)
    n110 = Not Equal?(x=w72, y=w105) -> (x != y?=w104:bool)
    n111 = case shown="真" w104 {
      tunnel: w72 -> [_ w254]
      tunnel: w99 -> [_ w261]
      tunnel: w98 -> [_ w260]
      frame False {
      }
      frame True {
        n112 = Subtract(x=w254, y=1) -> (x-y=w252:i32)
        "多列列表框" <- w252
        n113 = Subtract(x=w252, y=5) -> (x-y=w256:i32)
        n114 = property on="多列列表框" class="MCListbox (严格)"("ItemNames"=w261, "RowHdrs[]"=w260) -> (error out=w262:errorcluster)  [unwired: 2 in, 1 out]
        n115 = Greater Or Equal To 0?(x=w256) -> (x >= 0?=w255:bool)
        n116 = property on="多列列表框" class="MCListbox (严格)"(error in=w262) -> (error out=w263:errorcluster, "TopLeft"=w264:T12)  [unwired: 1 in, 1 out]
        n117 = Select(t=w256, s=w255, f=0) -> (s? t:f=w257:i32)
        n118 = Bundle By Name(cluster=w264, "Row"=w257) -> (w265:T12)
        n119 = property on="多列列表框" class="MCListbox (严格)"(error in=w263, "TopLeft"=w265) -> ()  [unwired: 1 in, 2 out]
      }
    }
  }
  n120 = property class="VI"(reference=w31) -> ("Name"=w30:string)  [unwired: 1 in, 2 out]
  n121 = call "总磷氨氮MB_api.vi"("STEP"=enum16{"open", "read", "write", "close"}."open") -> ("error out"=w7:errorcluster)  [unwired: 8 in, 2 out]
  n122 = Obtain Queue(name (unnamed)="NH3N" ("名称（未命名）"), element data type=cluster{"命令":string, "data":variant} {"命令"="", "data"=variant}) -> (queue out=w34:refnum<queue>, error out=w35:errorcluster)  [unwired: 3 in, 1 out]
  n123 = node-c288() -> (w5:T13)  [unwired: 4 in]
  n124 = property class="VI"(reference=w23) -> ("Name"=w16:string)  [unwired: 1 in, 2 out]
  n125 = control-ref of="测量模式下拉列表"() -> (w12:refnum<vi>)
  n126 = control-ref of="量程切换阈值"() -> (w10:refnum<vi>)
  n127 = control-ref of="参数下拉列表"() -> (w13:refnum<vi>)
  n128 = control-ref of="量程下拉列表"() -> (w14:refnum<vi>)
  n129 = timed-loop {
    timing: w5 -> [_]
    timing-out: [_] -> w4
    tunnel: w1 -> [w268]
    stop <- FALSE stop-if-true
    w269 = u16 3 items=["总磷"=1, "氨氮"=3] ("站号")
    # "定时更新"
    n130 = node-c288() -> ()  [unwired: 1 in, 1 out]
    n131 = call "总磷氨氮版本号读取.vi"() -> ("固件版本号"=→"固件版本号":string)  [unwired: 11 in]
    n132 = Bundle By Name(cluster=cluster{"命令":string, "data":variant} {"命令"="", "data"=variant} ("元素"), "命令"="读序列号", "data"=w269) -> (w267:cluster{"命令":string, "data":variant})
    n133 = Enqueue Element(queue=w268, element=w267) -> ()  [unwired: 2 in, 3 out]
    n134 = node-c288() -> ()  [unwired: 1 in, 1 out]
  }
  n135 = Open VI Reference(type specifier VI Refnum (for type only)=refnum<vi> refnum, vi path=w30, options=128 ("选项")) -> (vi reference=w28:refnum<vi>, error out=w26:errorcluster)  [unwired: 3 in]
  n136 = control-ref of="备用系数"() -> (w9:refnum<vi>)
  n137 = call-by-ref "?"(reference=w28, error in=w26) -> (reference out=w24:refnum<vi>, error out=w25:errorcluster)  [unwired: 12 in]
  n138 = control-ref of="公式"() -> (w11:refnum<vi>)
  n139 = Open VI Reference(type specifier VI Refnum (for type only)=refnum<vi> refnum, vi path=w16, options=128 ("选项")) -> (vi reference=w18:refnum<vi>, error out=w20:errorcluster)  [unwired: 3 in]
  n140 = Close Reference(reference=w24, error in (no error)=w25) -> ()  [unwired: 1 out]
  n141 = call-by-ref "?"(reference=w18, error in=w20) -> (reference out=w22:refnum<vi>, error out=w21:errorcluster)  [unwired: 12 in]
  n142 = while {
    tunnel: w34 -> [w277]
    shift-right: [w278] -> _
    shift-left: T4."待机" -> [w279]
    shift-right: [w275] -> _
    shift-left: u32 0 ("等待时间（毫秒）") -> [w276]
    stop <- FALSE stop-if-true
    n143 = Wait (ms)(milliseconds to wait=u32 1000 ("等待时间（毫秒）")) -> ()  [unwired: 1 out]
    n144 = local read "定时启动"() -> (w280:bool)
    n145 = case shown="真" w280 {
      tunnel: w279 -> [_ w288]
      tunnel: [T4."待机" w287] -> w278
      tunnel: w277 -> [_ w286]
      tunnel: w276 -> [_ w285]
      tunnel: [_ w284] -> w275
      frame False {
      }
      frame True {
        n146 = case shown="\"氨氮测量中\"" w288 {
          tunnel: [T4."启动氨氮" w293 w300 w311 w319 w331] -> w287
          tunnel: w286 -> [_ w298 _ w317 _ _]
          tunnel: w285 -> [_ _ _ _ _ w334]
          tunnel: [_ _ _ _ _ w330] -> w284
          frame "待机", Default {
          }
          frame "启动氨氮" {
            n147 = call "总磷氨氮启动命令.vi"("参数"=T16 {"站号"=3, "量程切换"=enum."AUTO", "控制命令"=enum."启动测量", "模式设置"=enum."待机", "测量间隔"=0}) -> ("启动命令"=w291:cluster{"命令":string, "data":variant})  [unwired: 10 in]
            n148 = Enqueue Element(queue=w298, element=w291) -> ()  [unwired: 2 in, 3 out]
            n149 = global read "VAR总磷氨氮全局变量.vi" "状态告警区"() -> (w297:T3)
            n150 = Unbundle By Name(w297) -> ("工作状态"=w296:T7)
            n151 = Not Equal To 0?(x=w296) -> (x != 0?=w295:bool)
            n152 = Select(t=T4."氨氮测量中", s=w295, f=T4."启动氨氮") -> (s? t:f=w293:T4)
          }
          frame "氨氮测量中" {
            n153 = flat-sequence {
              tunnel: [w304] -> w299
              tunnel: [w308] -> w300
              tunnel: w299 -> [w308]
              frame #0 {
                n154 = global read "VAR总磷氨氮全局变量.vi" "状态告警区"() -> (w305:T3)
                n155 = Unbundle By Name(w305) -> ("工作状态"=w306:T7)
                n156 = Equal To 0?(x=w306) -> (x = 0?=w301:bool)
                n157 = Select(t=T4."延时", s=w301, f=T4."氨氮测量中") -> (s? t:f=w304:T4)
              }
              frame #1 {
                n158 = Wait (ms)(milliseconds to wait=u32 5000 ("等待时间（毫秒）")) -> ()  [unwired: 1 out]
              }
            }
          }
          frame "启动总磷" {
            n159 = call "总磷氨氮启动命令.vi"("参数"=T16 {"站号"=1, "量程切换"=enum."AUTO", "控制命令"=enum."启动测量", "模式设置"=enum."待机", "测量间隔"=0}) -> ("启动命令"=w310:cluster{"命令":string, "data":variant})  [unwired: 10 in]
            n160 = Enqueue Element(queue=w317, element=w310) -> ()  [unwired: 2 in, 3 out]
            n161 = global read "VAR总磷氨氮全局变量.vi" "状态告警区"() -> (w312:T3)
            n162 = Unbundle By Name(w312) -> ("工作状态"=w313:T7)
            n163 = Not Equal To 0?(x=w313) -> (x != 0?=w314:bool)
            n164 = Select(t=T4."总磷测量中", s=w314, f=T4."启动总磷") -> (s? t:f=w311:T4)
          }
          frame "总磷测量中" {
            n165 = flat-sequence {
              tunnel: [w321] -> w318
              tunnel: [w327] -> w319
              tunnel: w318 -> [w327]
              frame #0 {
                n166 = global read "VAR总磷氨氮全局变量.vi" "状态告警区"() -> (w324:T3)
                n167 = Unbundle By Name(w324) -> ("工作状态"=w325:T7)
                n168 = Equal To 0?(x=w325) -> (x = 0?=w320:bool)
                n169 = Select(t=T4."延时", s=w320, f=T4."总磷测量中") -> (s? t:f=w321:T4)
              }
              frame #1 {
                n170 = Wait (ms)(milliseconds to wait=u32 5000 ("等待时间（毫秒）")) -> ()  [unwired: 1 out]
              }
            }
          }
          frame "延时" {
            n171 = local read "设置值"() -> (w333:dbl)
            n172 = Increment(x=w334) -> (x+1=w330:u32)
            n173 = Greater Or Equal?(x=w330, y=w333) -> (x >= y?=w332:bool)
            n174 = Select(t=T4."待机", s=w332, f=T4."延时") -> (s? t:f=w331:T4)
          }
        }
      }
    }
  }
  n175 = while {
    tunnel: w34 -> [w341]
    tunnel: w14 -> [w340]
    tunnel: w13 -> [w339]
    tunnel: w12 -> [w338]
    tunnel: w11 -> [w337]
    tunnel: w10 -> [w336]
    tunnel: w9 -> [w335]
    tunnel: w7 -> [_]
    stop <- FALSE stop-if-true
    n176 = event shown="[1] \"手动启动\": 值改变" {
      selector: _ -> [_ _ _ _ _ _ _ _ _ _ _ _ _ _ _]
      dyn-events: _ -> [_ _ _ _ _ _ _ _ _ _ _ _ _ _ _]
      timeout: _ -> [_ _ _ _ _ _ _ _ _ _ _ _ _ _ _]
      tunnel: w341 -> [_ w345 _ w356 w358 _ _ _ _ _ _ _ _ _ _]
      tunnel: w340 -> [_ _ _ _ _ _ _ _ _ w411 _ w431 w440 _ _]
      tunnel: w339 -> [_ _ _ _ _ _ _ _ _ w409 _ w429 w442 w450 w457]
      tunnel: w338 -> [_ _ _ _ _ _ _ _ _ w410 _ w430 w441 _ _]
      tunnel: w337 -> [_ _ _ _ _ _ _ _ _ w405 _ _ _ _ _]
      tunnel: w336 -> [_ _ _ _ _ _ _ _ _ _ _ w425 _ _ _]
      tunnel: w335 -> [_ _ _ _ _ _ _ _ _ _ _ _ _ w448 _]
      event Timeout {
        n177 = event-data() -> ()  [unwired: 1 in, 3 out]
      }
      event "手动启动": Value Change {
        n178 = event-data() -> ()  [unwired: 1 in, 6 out]
        n179 = call "总磷氨氮启动参数对话框.vi"() -> ("确认"=w343:bool, "元素"=w344:cluster{"命令":string, "data":variant})  [unwired: 10 in]
        n180 = case shown="真" w343 {
          tunnel: w345 -> [_ w347]
          tunnel: w344 -> [_ w346]
          frame False {
          }
          frame True {
            n181 = Enqueue Element(queue=w347, element=w346) -> ()  [unwired: 2 in, 3 out]
          }
        }
      }
      event "定时启动": Mouse Down {
        n182 = event-data() -> ()  [unwired: 1 in, 6 out]
        n183 = call "定时启动对话框.vi"() -> ("设置值"=→"设置值":dbl, "确定输出"=→"定时启动":bool)  [unwired: 10 in]
      }
      event "单步测试": Value Change {
        w351 = u16 1 items=["总磷"=1, "氨氮"=3] ("站号")
        n184 = event-data() -> ()  [unwired: 1 in, 6 out]
        n185 = Bundle("站号"=w351, "总磷氨氮调试"="总磷氨氮调试") -> (w350:cluster{"站号":u16, "总磷氨氮调试":u16[]})  [unwired: 1 in]
        n186 = Bundle By Name(cluster=cluster{"命令":string, "data":variant} {"命令"="", "data"=variant} ("元素"), "命令"="debug", "data"=w350) -> (w353:cluster{"命令":string, "data":variant})
        n187 = Enqueue Element(queue=w356, element=w353) -> ()  [unwired: 2 in, 3 out]
      }
      event "停止": Value Change {
        n188 = event-data() -> ()  [unwired: 1 in, 6 out]
        n189 = Enqueue Element(queue=w358, element=cluster{"命令":string, "data":variant} {"命令"="启动", "data"=variant(cluster{"站号":u16, "控制命令输出":u16[]} {"站号"=1, "控制命令输出"=[2816]})} ("元素")) -> ()  [unwired: 2 in, 3 out]
      }
      event "设置": Value Change {
        n190 = event-data() -> ()  [unwired: 1 in, 6 out]
        n191 = property on="窗格" class="Pane"("Origin"=T5 {"Horizontal"=0, "Vertical"=628} ("原点")) -> ()  [unwired: 2 in, 2 out]
      }
      event "返回": Value Change {
        n192 = event-data() -> ()  [unwired: 1 in, 6 out]
        n193 = property on="窗格" class="Pane"("Origin"=T5 {"Horizontal"=0, "Vertical"=0} ("原点")) -> ()  [unwired: 2 in, 2 out]
      }
      event "标液浓度1", "测量吸光度1", "测量吸光度2", "标液浓度2", "测量吸光度3", "标液浓度3", "测量吸光度4", "标液浓度4", "测量吸光度5", "标液浓度5", "样品1启用", "样品3启用", "样品4启用", "样品5启用", "样品2启用", "模型", "method", "样品1 F0", "样品1 F1", "样品2 F1", "样品2 F0", "样品3 F1", "样品4 F0", "样品4 F1", "样品5 F1", "样品5 F0", "精度": Value Change {
        n194 = event-data() -> ()  [unwired: 1 in, 6 out]
        n195 = formula code="E=log(F0/F1);"("F0"="样品1 F0", "F1"="样品1 F1") -> ("E"=w382:dbl)
        "测量吸光度1" <- w382
        n196 = formula code="E=log(F0/F1);"("F0"="样品2 F0", "F1"="样品2 F1") -> ("E"=w379:dbl)
        "测量吸光度2" <- w379
        n197 = formula code="E=log(F0/F1);"("F0"="样品3 F0", "F1"="样品3 F1") -> ("E"=w376:dbl)
        "测量吸光度3" <- w376
        n198 = formula code="E=log(F0/F1);"("F0"="样品4 F0", "F1"="样品4 F1") -> ("E"=w373:dbl)
        "测量吸光度4" <- w373
        n199 = formula code="E=log(F0/F1);"("F0"="样品5 F0", "F1"="样品5 F1") -> ("E"=w370:dbl)
        "测量吸光度5" <- w370
        n200 = Replace Array Subset(array=dbl[] [0.0, 0.0, 0.0, 0.0, 0.0] ("数组"), new element #1="标液浓度1", new element #2="标液浓度2", new element #3="标液浓度3", new element #4="标液浓度4", new element #5="标液浓度5") -> (w367:dbl[])  [unwired: 5 in]
        n201 = Replace Array Subset(array=dbl[] [0.0, 0.0, 0.0, 0.0, 0.0] ("数组"), new element #1=w382, new element #2=w379, new element #3=w376, new element #4=w373, new element #5=w370) -> (w366:dbl[])  [unwired: 5 in]
        n202 = Replace Array Subset(array=bool[] [FALSE, FALSE, FALSE, FALSE, FALSE] ("数组"), new element #1="样品1启用", new element #2="样品2启用", new element #3="样品3启用", new element #4="样品4启用", new element #5="样品5启用") -> (w365:bool[])  [unwired: 5 in]
        n203 = call "线性公式.vi"("精度"="精度", "模型"="模型", "method"="method", "启用"=w365, "监测浓度"=w366, "标液浓度"=w367) -> ("XY图"=→"XY图":cluster{"X Values":dbl[], "Y Values":dbl[]}[], "r^2"=→"r^2":dbl, "拟合方程"=→"拟合公式":string)  [unwired: 3 in]
      }
      event "标液浓度1", "标液浓度2", "标液浓度3", "标液浓度4", "标液浓度5", "样品1 F0", "样品1 F1", "样品2 F1", "样品2 F0", "样品3 F1", "样品3 F0", "样品4 F0", "样品4 F1", "样品5 F0", "样品5 F1", "精度", "公式.X^2", "公式.X", "公式.b", "量程切换阈值.阈值", "量程切换阈值.标液浓度", "备用系数.量程上限", "备用系数.量程下限", "备用系数.检出限", "备用系数.精度": Mouse Down {
        n204 = event-data() -> ("CtlRef"=w401:refnum<vi>)  [unwired: 1 in, 5 out]
        n205 = property class="DigNum (严格)"(reference=w401) -> (reference out=w399:refnum<vi>, "Value"=w400:dbl)  [unwired: 1 in, 1 out]
        n206 = call "数字键盘.vi"("OldNumber"=w400) -> ("NewNumber"=w398:sgl)
        n207 = property class="DigNum (严格)"(reference=w399, "Val(Sgnl)"=w398) -> ()  [unwired: 1 in, 2 out]
      }
      event "读公式": Value Change {
        n208 = event-data() -> ()  [unwired: 1 in, 6 out]
        n209 = property class="Enum (严格)"(reference=w409) -> ("Value"=w408:enum16{"氨氮", "总磷"})  [unwired: 1 in, 2 out]
        n210 = property class="Enum (严格)"(reference=w410) -> ("Value"=w407:enum16{"水样测量", "空白核查", "标样核查", "盲样测试", "加标回收"})  [unwired: 1 in, 2 out]
        n211 = property class="Enum (严格)"(reference=w411) -> ("Value"=w406:enum16{"低量程", "高量程"})  [unwired: 1 in, 2 out]
        n212 = call "总磷氨氮公式读取.vi"("量程"=w406, "测量模式"=w407, "测量参数"=w408) -> ("error out"=w403:errorcluster, "公式"=w404:cluster{"X^2":dbl, "X":dbl, "b":dbl})  [unwired: 7 in]
        n213 = property class="Clust (严格)"(reference=w405, "Value"=w404) -> ()  [unwired: 1 in, 2 out]
        n214 = case shown="错误" w403 {
          tunnel: ["读取成功" ("消息") "读取失败" ("消息")] -> w402
          frame No Error {
          }
          frame Error {
          }
        }
        n215 = One Button Dialog(message=w402) -> ()  [unwired: 1 in, 1 out]
      }
      event "写公式": Value Change {
        n216 = event-data() -> ()  [unwired: 1 in, 6 out]
        n217 = call "总磷氨氮公式写入.vi"("公式"="公式", "量程"="量程下拉列表", "测量模式"="测量模式下拉列表", "测量参数"="参数下拉列表") -> ("error out"=w414:errorcluster)  [unwired: 7 in]
        n218 = case shown="无错误" w414 {
          tunnel: ["写入成功" ("消息") "写入失败" ("消息")] -> w415
          frame No Error {
          }
          frame Error {
          }
        }
        n219 = One Button Dialog(message=w415) -> ()  [unwired: 1 in, 1 out]
      }
      event "量程切换阈值读取": Value Change {
        n220 = event-data() -> ()  [unwired: 1 in, 6 out]
        n221 = property class="Enum (严格)"(reference=w429) -> ("Value"=w428:enum16{"氨氮", "总磷"})  [unwired: 1 in, 2 out]
        n222 = property class="Enum (严格)"(reference=w430) -> ("Value"=w427:enum16{"水样测量", "空白核查", "标样核查", "盲样测试", "加标回收"})  [unwired: 1 in, 2 out]
        n223 = property class="Enum (严格)"(reference=w431) -> ("Value"=w426:enum16{"低量程", "高量程"})  [unwired: 1 in, 2 out]
        n224 = call "总磷氨氮量程读取.vi"("量程"=w426, "测量模式"=w427, "测量参数"=w428) -> ("error out"=w422:errorcluster, "量程切换阈值"=w424:cluster{"阈值":dbl, "标液浓度":dbl})  [unwired: 7 in]
        n225 = property class="Clust (严格)"(reference=w425, "Value"=w424) -> ()  [unwired: 1 in, 2 out]
        n226 = case shown="错误" w422 {
          tunnel: ["读取成功" ("消息") "读取失败" ("消息")] -> w423
          frame No Error {
          }
          frame Error {
          }
        }
        n227 = One Button Dialog(message=w423) -> ()  [unwired: 1 in, 1 out]
      }
      event "量程切换阈值写入": Value Change {
        n228 = event-data() -> ()  [unwired: 1 in, 6 out]
        n229 = property class="Enum (严格)"(reference=w442) -> ("Value"=w439:enum16{"氨氮", "总磷"})  [unwired: 1 in, 2 out]
        n230 = property class="Enum (严格)"(reference=w441) -> ("Value"=w438:enum16{"水样测量", "空白核查", "标样核查", "盲样测试", "加标回收"})  [unwired: 1 in, 2 out]
        n231 = property class="Enum (严格)"(reference=w440) -> ("Value"=w437:enum16{"低量程", "高量程"})  [unwired: 1 in, 2 out]
        n232 = call "总磷氨氮量程写入.vi"("量程切换阈值"="量程切换阈值", "量程"=w437, "测量模式"=w438, "测量参数"=w439) -> ("error out"=w434:errorcluster)  [unwired: 7 in]
        n233 = case shown="无错误" w434 {
          tunnel: ["写入成功" ("消息") "写入失败" ("消息")] -> w435
          frame No Error {
          }
          frame Error {
          }
        }
        n234 = One Button Dialog(message=w435) -> ()  [unwired: 1 in, 1 out]
      }
      event "备用系数读取": Value Change {
        n235 = event-data() -> ()  [unwired: 1 in, 6 out]
        n236 = property class="Enum (严格)"(reference=w450) -> ("Value"=w449:enum16{"氨氮", "总磷"})  [unwired: 1 in, 2 out]
        n237 = call "总磷氨氮备用系数读取.vi"("测量参数"=w449) -> ("error out"=w445:errorcluster, "备用系数"=w447:T1)  [unwired: 9 in]
        n238 = property class="Clust (严格)"(reference=w448, "Value"=w447) -> ()  [unwired: 1 in, 2 out]
        n239 = case shown="错误" w445 {
          tunnel: ["读取成功" ("消息") "读取失败" ("消息")] -> w446
          frame No Error {
          }
          frame Error {
          }
        }
        n240 = One Button Dialog(message=w446) -> ()  [unwired: 1 in, 1 out]
      }
      event "备用系数写入": Value Change {
        n241 = event-data() -> ()  [unwired: 1 in, 6 out]
        n242 = property class="Enum (严格)"(reference=w457) -> ("Value"=w456:enum16{"氨氮", "总磷"})  [unwired: 1 in, 2 out]
        n243 = call "总磷氨氮备用系数写入.vi"("备用系数"="备用系数", "测量参数"=w456) -> ("error out"=w453:errorcluster)  [unwired: 9 in]
        n244 = case shown="无错误" w453 {
          tunnel: ["写入成功" ("消息") "写入失败" ("消息")] -> w454
          frame No Error {
          }
          frame Error {
          }
        }
        n245 = One Button Dialog(message=w454) -> ()  [unwired: 1 in, 1 out]
      }
    }
  }
  n246 = while {
    tunnel: w34 -> [w475]
    tunnel: w35 -> [_]
    shift-right: [w469] -> _
    shift-left: enum16{"氨氮", "总磷"}."氨氮" ("枚举") -> [w470]
    stop <- FALSE stop-if-true
    w468 = u16 3 items=["总磷"=1, "氨氮"=3] ("站号")
    # "试剂填充 172 \n管路清洗108\n氨氮92\n总磷131\n总磷海水147\n总氮76\n总氮海水92"
    n247 = Wait (ms)(milliseconds to wait=u32 1000 ("等待时间（毫秒）")) -> ()  [unwired: 1 out]
    n248 = global read "VAR总磷氨氮全局变量.vi" "状态告警区"() -> (w466:T3)
    n249 = Bundle By Name(cluster=cluster{"命令":string, "data":variant} {"命令"="", "data"=variant} ("元素"), "命令"="读状态告警区", "data"=w468) -> (w477:cluster{"命令":string, "data":variant})
    n250 = Unbundle By Name(w466) -> ("系统时间"=w465:timestamp)
    n251 = Bundle By Name(cluster=cluster{"命令":string, "data":variant} {"命令"="", "data"=variant} ("元素"), "命令"="读测量数据区", "data"=w468) -> (w473:cluster{"命令":string, "data":variant})
    n252 = Enqueue Element(queue=w475, element=w477) -> (queue out=w471:refnum<queue>)  [unwired: 2 in, 2 out]
    n253 = Get Date/Time In Seconds() -> (seconds since 1Jan1904=w464:timestamp)
    n254 = Subtract(x=w464, y=w465) -> (x-y=w463:dbl)
    n255 = Enqueue Element(queue=w471, element=w473) -> (queue out=w467:refnum<queue>)  [unwired: 2 in, 2 out]
    n256 = Absolute Value(x=w463) -> (abs(x)=w462:dbl)
    n257 = Greater Or Equal?(x=w462, y=120.0) -> (x >= y?=w460:bool)
    n258 = case shown="真" w460 {
      tunnel: w467 -> [_ w482]
      frame False {
      }
      frame True {
        n259 = call "总磷氨氮启动命令.vi"("参数"=T17 {"站号"=3, "量程切换"=enum."AUTO", "控制命令"=enum."校时", "模式设置"=enum."待机", "测量间隔"=0}) -> ("启动命令"=w481:cluster{"命令":string, "data":variant})  [unwired: 10 in]
        n260 = Enqueue Element(queue=w482, element=w481) -> ()  [unwired: 2 in, 3 out]
      }
    }
    n261 = Increment(x=w470) -> (x+1=w469:enum16{"氨氮", "总磷"})
  }
  n262 = Close Reference(reference=w22, error in (no error)=w21) -> ()  [unwired: 1 out]
  n263 = node-c288(w4) -> ()  [unwired: 1 out]
